vi "Path.vi"() -> (2 "ini":path)   [LabVIEW 2016]
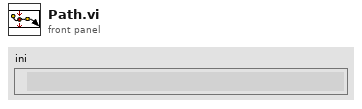
[diagram p1: front panel]
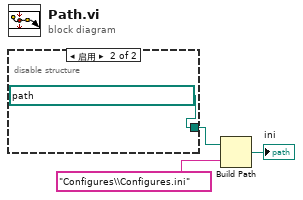
[diagram p0: block diagram]
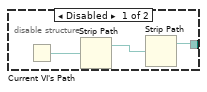
[diagram p2: hidden frame]
diagram:
  n1 = disable-structure shown="启用" {
    disable-tunnel: [w4 path "D:/SIEMENS/Code/PCB取料站"] -> w3
    frame Disabled {
      n2 = Current VI's Path() -> (path=w6:path)
      n3 = Strip Path(path=w6) -> (stripped path=w5:path)  [unwired: 1 out]
      n4 = Strip Path(path=w5) -> (stripped path=w4:path)  [unwired: 1 out]
    }
    frame Enabled {
    }
  }
  n5 = Build Path(base path=w3, name or relative path="Configures\\Configures.ini" ("名称或相对路径")) -> (appended path=→"ini":path)
